vi "Calib_Gas_Type.vi"(2 "Traverse line":T3 {"Row Duration (mins)" format="%#.1f"; "Row No" min=0; "Trace Gas Concentration (%)" min=0.0 format="%#_4f"; "Emission Rate (l/min)" format="%#.2f"; "Tunnel Speed" format="%#.2f"; "Start X" format="%#.2f"; "Start Y" format="%#.2f"; "Start Z" format="%#.2f"; "End X" format="%#.2f"; "End Y" format="%#.2f"; "End Z" format="%#.2f"; "Averaging time (min)" min=0.0 format="%#.2f"}, 3 "Simulate/Run":T2, 4 "Requested Position":T1=1 items=["Zero Air", "Calib 1", "Calib 2", "Measure"]) -> (0 "Traverse line Out":T3 {"Row Duration (mins)" format="%#.1f"; "Row No" min=0; "Trace Gas Concentration (%)" min=0.0 format="%#_4f"; "Emission Rate (l/min)" format="%#.2f"; "Tunnel Speed" format="%#.2f"; "Start X" format="%#.2f"; "Start Y" format="%#.2f"; "Start Z" format="%#.2f"; "End X" format="%#.2f"; "End Y" format="%#.2f"; "End Z" format="%#.2f"; "Averaging time (min)" min=0.0 format="%#.2f"}, 1 "Requested Position Out":T1=1 items=["Zero Air", "Calib 1", "Calib 2", "Measure"])   [LabVIEW 2014]
uses:
  Gen Trav/Traverse_cluster.ctl
  Gen Trav/Spacing.ctl
  Controls/Multi_run_mode.ctl
  ADAM Client/Sub VIs/ADAM Controls/Valco_valve_ph.ctl
  Controls/User_Specific_mode.ctl
panel:
  # "X           Y            Z"
  # "Start"
  # "End"
  # "X           Y            Z"
  # "Start"
  # "End"
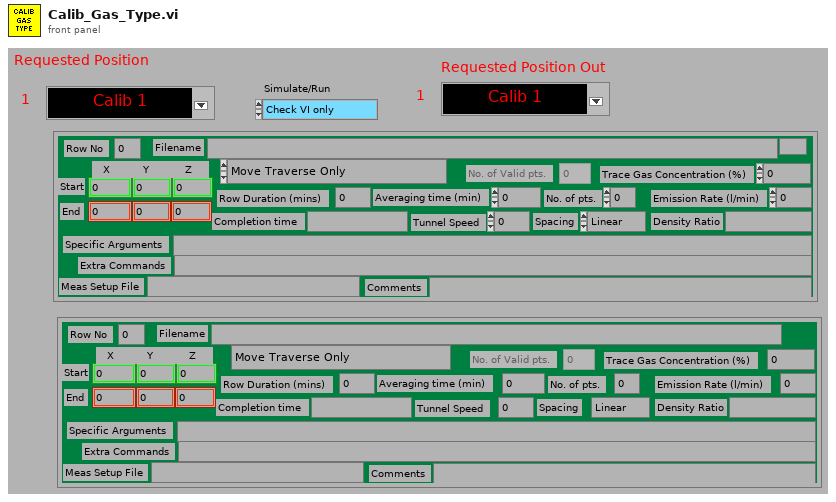
[diagram p1: front panel]
types:
  T1 = typedef "Valco_valve_ph.ctl" = u16
  T2 = typedef "User_Specific_mode.ctl" = enum16{"Check VI only", "Run VI"}
  T3 = typedef "Traverse_cluster.ctl" = cluster{"Start X":dbl, "Start Y":dbl, "Start Z":dbl, "End X":dbl, "End Y":dbl, "End Z":dbl, "No. of pts.":i32, "Spacing":T4, "Filename":path, "Tunnel Speed":dbl, "Averaging time (min)":dbl, "Extra Commands":string, "Specific Arguments":string, "Emission Rate (l/min)":dbl, "Trace Gas Concentration (%)":dbl, "Density Ratio":string, "Comments":string, "Row No":i32, "Row Type Selector":T5, "Completion time":string, "Row Duration (mins)":dbl, "No. of Valid pts.":i32, "Meas Setup File":string}
  T4 = typedef "Spacing.ctl" = enum16{"Linear", "Log", "Gauss", "Specified", "N/A"}
  T5 = typedef "Multi_run_mode.ctl" = enum16{"Move Traverse Only", "Set Tunnel Speed Only", "Set Source Only", "Set Measurement Conditions", "Single Measurement", "Vertical Profile", "Lateral Profile", "Longitudinal Profile", "Explore Volume", "Multi-Axis Profile", "Auto Calibrate", "Meas Fast FID Bkgnd", "Check Beam Power", "Scanning Valve Measurement", "Run VI Named:", "Set ADAM Ch", "Wait (minutes)", "Send Message", "Synchronize With:", "Fall Back to this Row", "Turn Off Row Repeating", "Blank Row", "Traverse 3D Volume"}
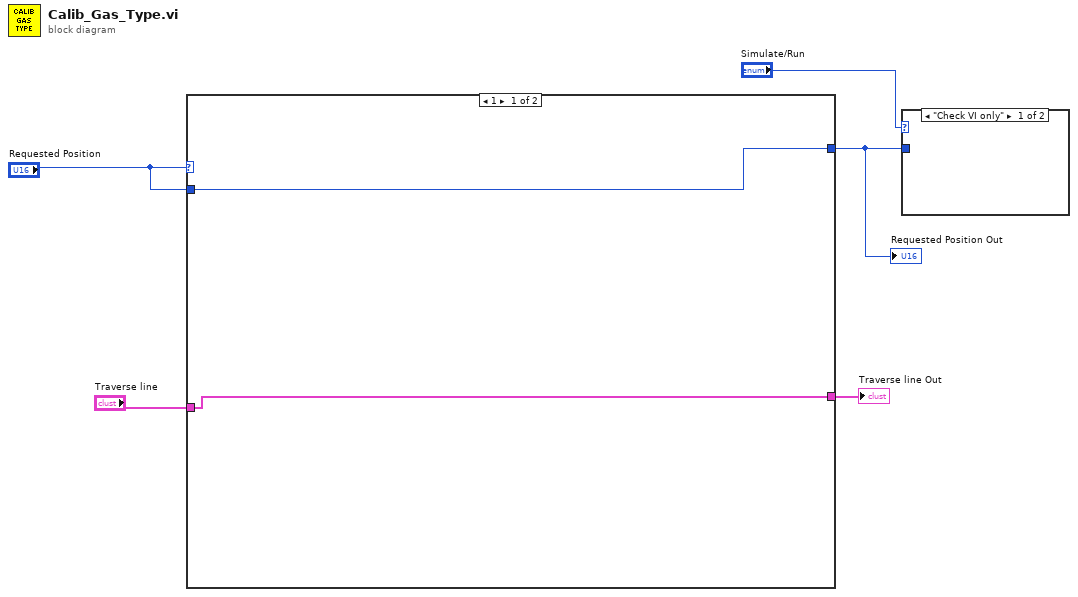
[diagram p0: block diagram]
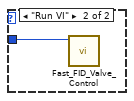
[diagram p2: hidden frame]
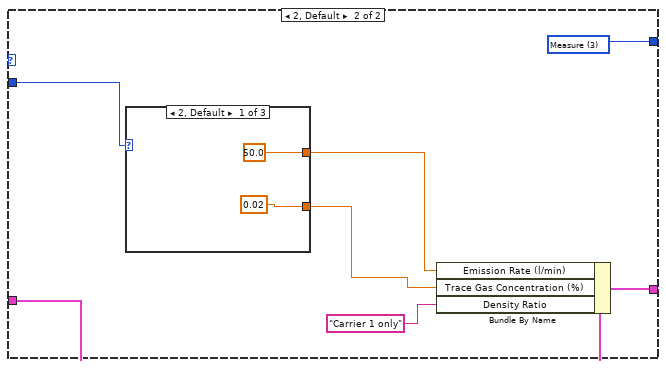
[diagram p3: hidden frame]
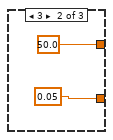
[diagram p4: hidden frame]
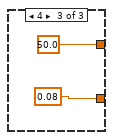
[diagram p5: hidden frame]
diagram:
  n1 = case shown="1" "Requested Position" {
    tunnel: [w7 w14] -> w5
    tunnel: "Traverse line" -> [w7 w13]
    tunnel: "Requested Position" -> [w6 w12]
    tunnel: [w6 w8] -> w2
    frame 1 {
    }
    frame 2, Default {
      w8 = T1 3 items=["Zero Air", "Calib 1", "Calib 2", "Measure"] ("Requested Position")
      n2 = case shown="2, Default" w12 {
        tunnel: [50.0 ("Emission Rate (l/min)") 50.0 ("Emission Rate (l/min)") 50.0 ("Emission Rate (l/min)")] -> w10
        tunnel: [0.02 ("Trace Gas Concentration (%)") 0.05 ("Trace Gas Concentration (%)") 0.08 ("Trace Gas Concentration (%)")] -> w9
        frame 2, Default {
        }
        frame 3 {
        }
        frame 4 {
        }
      }
      n3 = Bundle By Name(cluster=w13, "Emission Rate (l/min)"=w10, "Trace Gas Concentration (%)"=w9, "Density Ratio"="Carrier 1 only") -> (w14:T3)
    }
  }
  "Traverse line Out" <- w5
  "Requested Position Out" <- w2
  n4 = case shown="\"Check VI only\"" "Simulate/Run" {
    tunnel: w2 -> [_ w21]
    frame "Check VI only" {
    }
    frame "Run VI" {
      n5 = call "Fast_FID_Valve_Control.vi"("Requested Position"=w21) -> ()  [unwired: 7 out]
    }
  }
